vi "Break Diagram.vi"   [LabVIEW 2024, in "Utilities.lvlib"]
uses:
  Utilities.lvlib
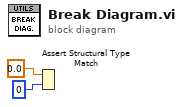
[diagram p0: block diagram]
diagram:
  n1 = Assert Structural Type Match(0:0, 1:0.0) -> ()
